vi "coerce and update control.vi"(8 "error in (no error)":errorcluster, 9 "max (+Inf)":dbl=inf, 10 "min (-Inf)":dbl=-inf, 11 "Refnum In":refnum<vi>) -> (0 "error out":errorcluster, 2 "Value":dbl, 3 "Copy Refnum Out":refnum<vi>)   [LabVIEW 2020]
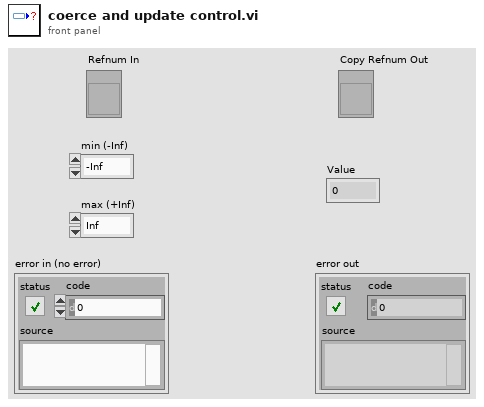
[diagram p1: front panel]
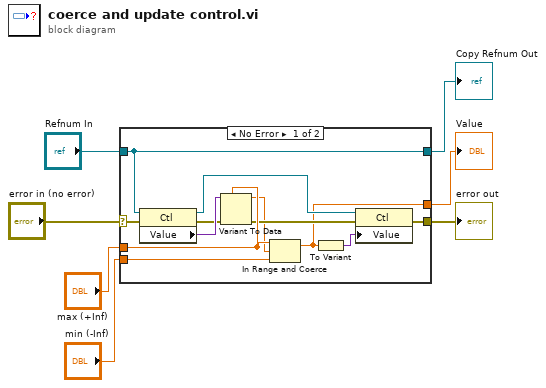
[diagram p0: block diagram]
diagram:
  n1 = case shown="No Error" "error in (no error)" {
    selector: "error in (no error)" -> [w18 w22]
    tunnel: [w16 w22] -> w6
    tunnel: [w19 w21] -> w5
    tunnel: "Refnum In" -> [w19 w21]
    tunnel: "min (-Inf)" -> [w15 w20]
    tunnel: "max (+Inf)" -> [w13 _]
    tunnel: [w8 w20] -> w1
    frame No Error {
      n2 = property class="Ctl"(reference=w19, error in=w18) -> (reference out=w17:refnum<vi>, error out=w12:errorcluster, "Value"=w14:variant)
      n3 = Variant To Data(error in=w12, type=w13, Variant=w14) -> (data=w10:dbl, error out=w11:errorcluster)
      n4 = In Range and Coerce(upper limit=w13, x=w10, lower limit=w15) -> (coerced(x)=w8:dbl)  [unwired: 1 out]
      n5 = To Variant(anything=w8) -> (Variant=w9:variant)
      n6 = property class="Ctl"(reference=w17, error in=w11, "Value"=w9) -> (error out=w16:errorcluster)  [unwired: 1 out]
    }
    frame Error {
    }
  }
  "Copy Refnum Out" <- w5
  "error out" <- w6
  "Value" <- w1
